vi "Clase7b.vi"() -> ()   [LabVIEW 2011]
panel:
  out "Contador":dbl
  out "Menor":dbl
  out "Mayor":dbl
  out "Promedio":dbl
  out "Temperatura":i32(slide) scale=0.0..100.0
  # "Generar (10 temperaturas) y al final presentar la temperatura mayor, menor y la temperatura promedio"
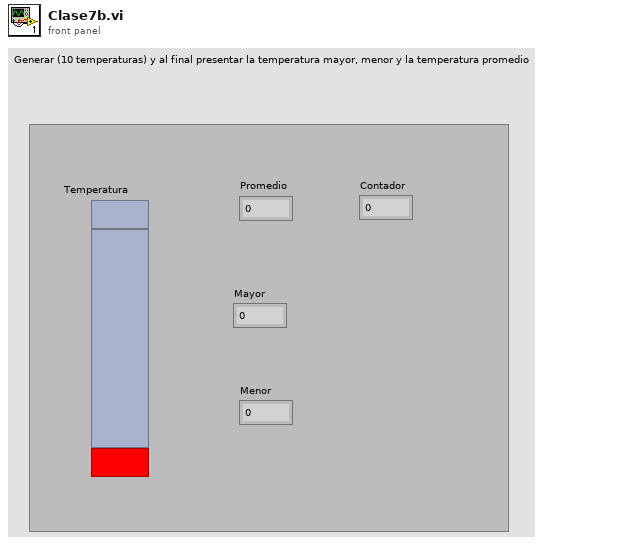
[diagram p1: front panel]
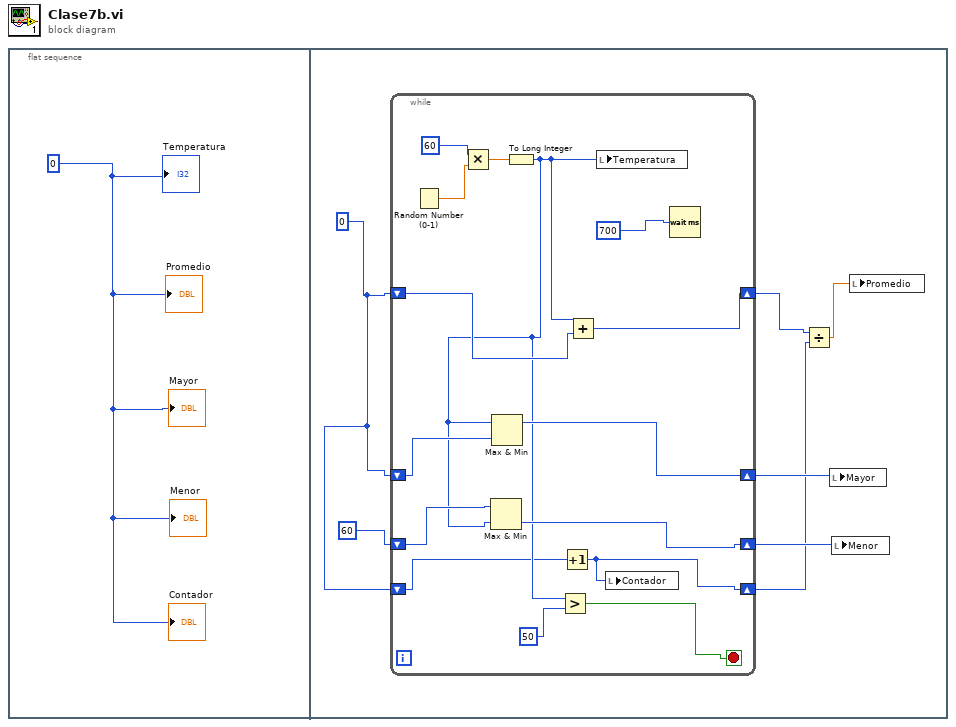
[diagram p0: block diagram]
diagram:
  n1 = flat-sequence {
    frame #0 {
      w1 = 0
      "Temperatura" <- w1
      "Promedio" <- w1
      "Mayor" <- w1
      "Menor" <- w1
      "Contador" <- w1
    }
    frame #1 {
      w3 = 0
      n2 = while {
        shift-right: [w19] -> w8
        shift-left: w3 -> [w20]
        shift-right: [w16] -> w6
        shift-left: w3 -> [w17]
        shift-right: [w14] -> w5
        shift-left: 60 -> [w15]
        shift-right: [w9] -> w2
        shift-left: w3 -> [w10]
        stop <- w11 stop-if-true
        n3 = Random Number (0-1)() -> (number: 0 to 1=w21:dbl)
        n4 = Multiply(x=60, y=w21) -> (x*y=w23:dbl)
        n5 = To Long Integer(number=w23) -> (32bit integer=w12:i32)
        n6 = Max & Min(x=w15, y=w12) -> (min(x,y)=w14:i32)  [unwired: 1 out]
        n7 = Max & Min(x=w12, y=w17) -> (max(x,y)=w16:i32)  [unwired: 1 out]
        n8 = Greater?(x=w12, y=50) -> (0:w11:bool)
        n9 = Increment(x=w10) -> (x+1=w9:i32)
        n10 = Add(x=w12, y=w20) -> (x+y=w19:i32)
        n11 = local write "Temperatura"(w12) -> ()
        n12 = local write "Contador"(w9) -> ()
        n13 = Wait (ms)(milliseconds to wait=700) -> ()  [unwired: 1 out]
      }
      n14 = Divide(x=w8, y=w2) -> (x/y=w7:dbl)
      n15 = local write "Mayor"(w6) -> ()
      n16 = local write "Menor"(w5) -> ()
      n17 = local write "Promedio"(w7) -> ()
    }
  }
